vi "04T_service_byte_Parsing.vi"(11 "Service Byte":u8) -> (2 "Flags":T1, 3 "Green LED":bool)   [LabVIEW 2013]
panel:
  out "Heating":bool
  out "Heater\nEnabled":bool
  out "Ramping":bool
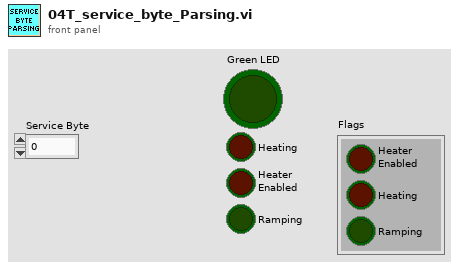
[diagram p1: front panel]
types:
  T1 = cluster{"Heater\nEnabled":bool, "Heating":bool, "Ramping":bool}
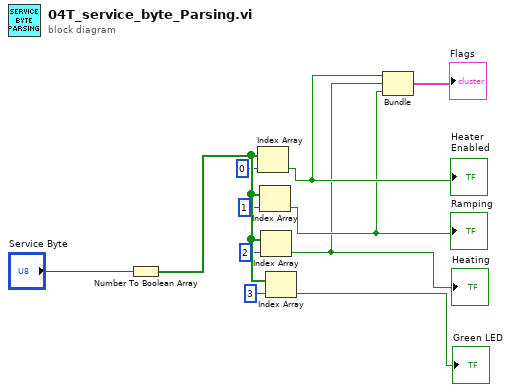
[diagram p0: block diagram]
diagram:
  n1 = Number To Boolean Array(number="Service Byte") -> (Boolean array=w11:bool[])
  n2 = Index Array(array=w11, index=0) -> (element=w3:bool)
  "Heater\nEnabled" <- w3
  n3 = Index Array(array=w11, index=1) -> (element=w2:bool)
  "Ramping" <- w2
  n4 = Index Array(array=w11, index=2) -> (element=w1:bool)
  "Heating" <- w1
  n5 = Index Array(array=w11, index=3) -> (element=→"Green LED":bool)
  n6 = Bundle(w3, w1, w2) -> (→"Flags":cluster{bool, bool, bool})  [unwired: 1 in]
